vi "CAlex2_Display.vi"(4 "AnkleTraj_Target":dbl[][](array[numeric])=[[0.24613333333333332, -0.7388833333333333, 0.0], [0.24515578259561696, -0.7391742724681776, 0.0], [0.24429789520875214, -0.739459405874052, 0.0], [0.24448752074226363, -0.7393345947088731, 0.0], [0.24469655916514985, -0.7392478031578622, 0.0], [0.24405664388628898, -0.7394239868907534, 0.0], [0.24328071991783762, -0.7396182885443063, 0.0], [0.2423466978742433, -0.7400415973949248, 0.0], [0.24125052807279473, -0.7405823353848426, 0.0], [0.24023250332483256, -0.7409537571683317, 0.0], [0.23967630694566833, -0.7410411536139305, 0.0], [0.2384997454338211, -0.7415221213338982, 0.0], [0.23592724691682573, -0.7427406041862703, 0.0], [0.2344645352495657, -0.7433585608236463, 0.0], [0.2332252795319526, -0.7437143391621577, 0.0], [0.2327208992774311, -0.7438576185144828, 0.0], [0.22915465606710558, -0.7454581765152355, 0.0], [0.2268128238804998, -0.7463847644792208, 0.0], [0.22529565802150417, -0.7469229398096506, 0.0], [0.2250314142391736, -0.7469447859134761, 0.0], [0.22156812672606813, -0.7483363962699071, 0.0], [0.21883255251595407, -0.7494578681789847, 0.0], [0.21756136754091762, -0.7498326608958199, 0.0], [0.2168187315034995, -0.7500358029214264, 0.0], [0.21497895218156837, -0.7506468649505054, 0.0], [0.21286079288286486, -0.7514266489532438, 0.0], [0.21166342103005523, -0.751737076640361, 0.0], [0.21054528432667385, -0.7520154789594069, 0.0], [0.2095433751260343, -0.7522629402601544, 0.0], [0.20845287441942323, -0.752488930880239, 0.0], [0.20742095365351557, -0.752704190462103, 0.0], [0.2051133246644528, -0.753343768184596, 0.0], [0.2038687493698828, -0.7536810637153099, 0.0], [0.2017501089727274, -0.754314257743821, 0.0], [0.19969644651868348, -0.7547514921885444, 0.0], [0.19826758992028087, -0.7551034048067478, 0.0], [0.19615360503043353, -0.7556945908696338, 0.0], [0.19343486835440665, -0.7565103575172124, 0.0], [0.19053313834169708, -0.7574473371460267, 0.0], [0.18843960759791628, -0.7580404798772611, 0.0], [0.18644089773884542, -0.7586060395277501, 0.0], [0.18390809075480052, -0.7594539816458029, 0.0], [0.1808701460626755, -0.7604695651212671, 0.0], [0.17793764820403346, -0.7614543964796003, 0.0], [0.1767810377685385, -0.7618396967115929, 0.0], [0.17456520772270492, -0.7625875498088734, 0.0], [0.17246929355256413, -0.7633236532400511, 0.0], [0.17065935181250597, -0.763955274420301, 0.0], [0.16925675895803116, -0.7643810549322506, 0.0], [0.1685767951889886, -0.7646594472602406, 0.0], [0.16694206859877006, -0.7652765726365656, 0.0], [0.1657034054333985, -0.7656183932135866, 0.0], [0.16450452568282725, -0.7660516442264967, 0.0], [0.1643715030160247, -0.7661069672108636, 0.0], [0.1625504624989272, -0.7667395140519705, 0.0], [0.1616783617927418, -0.7669891645306469, 0.0], [0.16033780666677916, -0.76741690328083, 0.0], [0.16006736860588602, -0.7674978448523857, 0.0], [0.15831402282464435, -0.7680654888349482, 0.0], [0.15675268420907598, -0.768505933121761, 0.0], [0.15526824545197823, -0.7689202252501333, 0.0], [0.1541607197723348, -0.7692489433810146, 0.0], [0.15245036106216156, -0.7696931341913663, 0.0], [0.14957434419557783, -0.7704715732684904, 0.0], [0.14828391270870533, -0.7707643989263094, 0.0], [0.14559288612896337, -0.7714308621646974, 0.0], [0.14439132840557845, -0.7717045322626312, 0.0], [0.1403678029587542, -0.7726695796663579, 0.0], [0.13890481051768733, -0.7729677173493494, 0.0], [0.13575718504559817, -0.7736433469259514, 0.0], [0.1343570726368564, -0.7739458151834464, 0.0], [0.13099009466893163, -0.774589891801166, 0.0], [0.12911814969929047, -0.774937273450445, 0.0], [0.12611842200944545, -0.7754845226684387, 0.0], [0.12384219776075701, -0.7759407221358413, 0.0], [0.12069834992424777, -0.7764745331284479, 0.0], [0.118341694530081, -0.7768570378169698, 0.0], [0.11607436638610731, -0.7772018607169953, 0.0], [0.11314798387040843, -0.7777047090591378, 0.0], [0.11050956015431135, -0.7781152538350306, 0.0], [0.10756675505982971, -0.778548547769883, 0.0], [0.10601252580438528, -0.77874213616469, 0.0], [0.10300893051989053, -0.7791434222500895, 0.0], [0.10059842214669534, -0.7794940247796804, 0.0], [0.09745929116516489, -0.7798971713729205, 0.0], [0.09629140586409997, -0.7800241310447404, 0.0], [0.09332400376079654, -0.780333694859322, 0.0], [0.09103242965898439, -0.7806270861703188, 0.0], [0.08770797963904334, -0.7809774861562493, 0.0], [0.08659441058384258, -0.7810698580287234, 0.0], [0.08426991411154908, -0.7812735166409136, 0.0], [0.0818464656125101, -0.781542090954264, 0.0], [0.07860913641931493, -0.7818772944590949, 0.0], [0.07707091026740395, -0.7820113723411644, 0.0], [0.07555596720741292, -0.7821230905218299, 0.0], [0.07305848865222275, -0.7823716410535728, 0.0], [0.07035157530401719, -0.782669419508252, 0.0], [0.06826387205643206, -0.782862017318102, 0.0], [0.0674716614358491, -0.7829060320001467, 0.0], [0.06506043561731781, -0.7831504929572028, 0.0], [0.06310157689899608, -0.7833812806557202, 0.0], [0.060651473518367305, -0.7836169696991431, 0.0], [0.06010231092573205, -0.7836307056693828, 0.0], [0.05848974929547346, -0.7837615507718494, 0.0], [0.05697455308933186, -0.7839656398243741, 0.0], [0.05464840918973575, -0.7842448590639965, 0.0], [0.05398829908766164, -0.7842628754609134, 0.0], [0.05284711042908441, -0.784307967671166, 0.0], [0.05184067068631544, -0.7844328724163524, 0.0], [0.05004952975847894, -0.7846922419674446, 0.0], [0.04917933101630442, -0.7847515944572329, 0.0], [0.0482067357714643, -0.7847515052312516, 0.0], [0.04700591000093282, -0.784863011448222, 0.0], [0.045323652125186624, -0.78512585869287, 0.0], [0.04441352388868794, -0.7852503533177574, 0.0], [0.04358011009025365, -0.7852037874533097, 0.0], [0.0424444654208676, -0.7852875753729346, 0.0], [0.04126004570310824, -0.7855186232616822, 0.0], [0.040124937873396105, -0.7857250610546572, 0.0], [0.03947411689805993, -0.7856815785943572, 0.0], [0.03845736540920874, -0.7856700898215838, 0.0], [0.037603444107991116, -0.785821981733852, 0.0], [0.03668912531087186, -0.7860330270037836, 0.0], [0.03631201610250871, -0.7860165362475472, 0.0], [0.03522455718085865, -0.7859789899374554, 0.0], [0.03474142561323009, -0.7860480904168305, 0.0], [0.03415715660823453, -0.7862604703380354, 0.0], [0.03381691913063367, -0.7862910817190454, 0.0], [0.03292340364750774, -0.7862265024447485, 0.0], [0.03241768234328942, -0.7862481196110391, 0.0], [0.03202665488082627, -0.7864321951305296, 0.0], [0.03182900463295782, -0.7865167784204048, 0.0], [0.031079149209339147, -0.7864808831658114, 0.0], [0.03038515590143912, -0.7864844060803323, 0.0], [0.030159588775692234, -0.7865929996865106, 0.0], [0.029889439890187133, -0.7867169560834536, 0.0], [0.029348085042040933, -0.7867009127262867, 0.0], [0.028561668290352536, -0.7866845556438959, 0.0], [0.028189689874212, -0.7867619987382084, 0.0], [0.027745017070139672, -0.786942964387257, 0.0], [0.027362567657518766, -0.7869644614468956, 0.0], [0.02638692892411661, -0.7869626934102248, 0.0], [0.026068754674981046, -0.7869979402918131, 0.0], [0.02517144759700583, -0.7872004163901596, 0.0], [0.02477784012412534, -0.7872491344056932, 0.0], [0.02383566271078354, -0.7872600104612801, 0.0], [0.02348938288371493, -0.7872789034032597, 0.0], [0.022213703173392288, -0.7874720576093395, 0.0], [0.021651810632390148, -0.7875615394086567, 0.0], [0.02072286196310254, -0.7875726828739505, 0.0], [0.020294470227114565, -0.7875725727644182, 0.0], [0.019039907077098052, -0.7877057059014416, 0.0], [0.01765463045533501, -0.7878660774364988, 0.0], [0.017008568231705417, -0.7878705475875676, 0.0], [0.016331238534833797, -0.7878674577459974, 0.0], [0.015301524598534443, -0.7879500971410542, 0.0], [0.013175004264126587, -0.7881227684994365, 0.0], [0.012599532933974972, -0.7881362882774775, 0.0], [0.011590794788298088, -0.7881326595475248, 0.0], [0.010982212566540302, -0.7881624877206551, 0.0], [0.008430877492632908, -0.7883089958216887, 0.0], [0.0073701656804433385, -0.7883637054459357, 0.0], [0.006534401238598057, -0.7883369603305339, 0.0], [0.005857106769173521, -0.7883408246568849, 0.0], [0.0036341933158762904, -0.7884203918373144, 0.0], [0.0017199396753864325, -0.7885010154094342, 0.0], [0.001054794556211927, -0.7884804659115676, 0.0], [0.0002567263877230023, -0.7884729911380082, 0.0], [-0.0013181108486029758, -0.7884919168187614, 0.0], [-0.004009114624084201, -0.7885646159414788, 0.0], [-0.004721619017951035, -0.788563571578087, 0.0], [-0.005490707534985728, -0.7885368856950778, 0.0], [-0.006720271622264472, -0.7885221798013166, 0.0], [-0.00946256190968962, -0.7885426790574998, 0.0], [-0.0107773510970461, -0.7885526806198543, 0.0], [-0.011404177158667525, -0.7885254499937199, 0.0], [-0.01230370632954732, -0.7885099737771037, 0.0], [-0.014783720031384435, -0.788505360160213, 0.0], [-0.016655495616472324, -0.7885000050444746, 0.0], [-0.017352058861391, -0.7884684140217153, 0.0], [-0.01801104065566522, -0.7884278820318243, 0.0], [-0.020159474340736516, -0.7883818273511758, 0.0], [-0.022198356752492057, -0.7883834862202718, 0.0], [-0.023377406887171867, -0.7883564009689698, 0.0], [-0.023715126260462696, -0.7883258761914703, 0.0], [-0.02546803605106259, -0.7882808163999377, 0.0], [-0.02764678331393335, -0.7882522527772768, 0.0], [-0.02900583751499738, -0.7882179655472195, 0.0], [-0.029503264776825258, -0.7881835478310103, 0.0], [-0.030670043396237794, -0.7881356235738904, 0.0], [-0.03290540286290335, -0.7880696389206449, 0.0], [-0.03424051453549059, -0.7880319431567786, 0.0], [-0.03518867698164292, -0.7879865813917275, 0.0], [-0.035708520712345156, -0.7879516963423487, 0.0], [-0.03785604851305007, -0.7878534552815656, 0.0], [-0.039173831000815784, -0.7878079902289162, 0.0], [-0.04031305495094807, -0.7877480464957666, 0.0], [-0.040775374063418565, -0.7877090222363465, 0.0], [-0.042371807747924595, -0.7876329980068867, 0.0], [-0.04390308424613412, -0.7875610592614354, 0.0], [-0.044893376222619144, -0.7875144179579441, 0.0], [-0.04564564925107059, -0.7874679571001013, 0.0], [-0.04656707813226394, -0.7874055062676626, 0.0], [-0.04824029119510185, -0.7872916822301301, 0.0], [-0.04904894550139232, -0.7872516191181922, 0.0], [-0.05000363023846826, -0.7871794139623552, 0.0], [-0.05069263439155017, -0.7871412478324679, 0.0], [-0.05202764767163273, -0.7870474284270107, 0.0], [-0.05298811443341366, -0.7869667161446681, 0.0], [-0.053770878548014114, -0.7868941577787267, 0.0], [-0.05459432155515526, -0.7868264205955833, 0.0], [-0.055461819619422065, -0.7867529685001882, 0.0], [-0.056634066465346904, -0.7866465700876712, 0.0], [-0.057223819714484835, -0.7865958266471488, 0.0], [-0.05822818983782874, -0.7864995542146789, 0.0], [-0.05888556085452924, -0.7864434159578955, 0.0], [-0.05997878318995532, -0.786336537681881, 0.0], [-0.060747251544050335, -0.7862651717599778, 0.0], [-0.06154929157510758, -0.7861805478817437, 0.0], [-0.06238461562291835, -0.7860944181250622, 0.0], [-0.06321052646340114, -0.7860077538688077, 0.0], [-0.06431083300249688, -0.7858786867171308, 0.0], [-0.0649946346567653, -0.7858022812056326, 0.0], [-0.06597802816340989, -0.7856949410158913, 0.0], [-0.06663767976420029, -0.7856173886891471, 0.0], [-0.06795606111781928, -0.7854548450334109, 0.0], [-0.06885321364907762, -0.785351471611811, 0.0], [-0.06967376061251168, -0.7852434997192976, 0.0], [-0.0706422839266972, -0.7851287975124323, 0.0], [-0.07166185154535253, -0.7850070449374327, 0.0], [-0.07320001399122117, -0.7848166996970609, 0.0], [-0.07366284492618107, -0.7847477237306885, 0.0], [-0.07509107248592095, -0.7845846675065444, 0.0], [-0.07573304869493647, -0.7844933210836742, 0.0], [-0.07783852524090834, -0.7841811413409909, 0.0], [-0.07830638873019802, -0.784113816047286, 0.0], [-0.07986142248668965, -0.7839136830476261, 0.0], [-0.08057983843469357, -0.7838133611250357, 0.0], [-0.08254712925686795, -0.7835107319583848, 0.0], [-0.08372130434764231, -0.7833332506546589, 0.0], [-0.08487482140537983, -0.783178322028624, 0.0], [-0.08624135215637413, -0.7830037405553079, 0.0], [-0.08748571040426449, -0.7827962829871418, 0.0], [-0.0895638539320319, -0.7824591761767064, 0.0], [-0.09033022919915192, -0.7823437713500916, 0.0], [-0.09223469613748583, -0.7820558585723796, 0.0], [-0.09303631599513518, -0.7819242041034085, 0.0], [-0.09537564242715288, -0.7814955495412113, 0.0], [-0.09647386843985803, -0.781298844845439, 0.0], [-0.0983505446047384, -0.7809952024764676, 0.0], [-0.09939197545609449, -0.7808303999018062, 0.0], [-0.10117703859613394, -0.780479144010592, 0.0], [-0.10307739897768062, -0.7801058716544537, 0.0], [-0.10458410669158132, -0.7798233513601808, 0.0], [-0.10631614948309831, -0.7795040320845944, 0.0], [-0.10724061359126007, -0.7793124203492745, 0.0], [-0.1098252331880692, -0.7787507023360662, 0.0], [-0.11118802584963487, -0.7784571826812104, 0.0], [-0.1134401070088136, -0.7780001641140143, 0.0], [-0.11398997768348407, -0.7778998615960213, 0.0], [-0.1164778575110416, -0.7772996866609776, 0.0], [-0.1181717940663653, -0.7768863467573213, 0.0], [-0.12066860475959379, -0.7763223189444195, 0.0], [-0.1214141962112577, -0.7761766991536709, 0.0], [-0.12324044731997584, -0.7756735262994104, 0.0], [-0.1254773206809978, -0.7750478230549499, 0.0], [-0.1278924360774777, -0.7744240727286277, 0.0], [-0.12921853695853153, -0.7741273427918501, 0.0], [-0.13026599200310643, -0.7738321755872171, 0.0], [-0.1328264905613512, -0.7730393629477945, 0.0], [-0.13517221445668215, -0.772357930314364, 0.0], [-0.13720511623991974, -0.7718098114576666, 0.0], [-0.13770659806181337, -0.771675739116628, 0.0], [-0.1401844389971911, -0.7708316127409436, 0.0], [-0.14248754289563006, -0.7700929873871858, 0.0], [-0.14503768099654107, -0.769289278577148, 0.0], [-0.14557750618101167, -0.7691803977996958, 0.0], [-0.14746986736043616, -0.7684261182538246, 0.0], [-0.14991232932304877, -0.7675411849979178, 0.0], [-0.1525093218513537, -0.7666150255659575, 0.0], [-0.15352826964278496, -0.7663174796823413, 0.0], [-0.15462071853739745, -0.7658054188771892, 0.0], [-0.1572225876287715, -0.7647397773653982, 0.0], [-0.15956896179024835, -0.7638012789023148, 0.0], [-0.16118181666413148, -0.7631848529453348, 0.0], [-0.1617132790024308, -0.7629132233699157, 0.0], [-0.16400798872387004, -0.7617854289722976, 0.0], [-0.16614694592442525, -0.7608493885441028, 0.0], [-0.16794638606264142, -0.7599932650782975, 0.0], [-0.1683225857071199, -0.759779362579468, 0.0], [-0.1699769170071399, -0.7587593491288297, 0.0], [-0.17186490276842684, -0.7577711398641326, 0.0], [-0.17349617867901543, -0.7567964031229927, 0.0], [-0.17392368788780974, -0.7564718113150823, 0.0], [-0.17491070255363497, -0.7556716244470942, 0.0], [-0.17651750620363071, -0.7545597916249724, 0.0], [-0.17799167744774833, -0.7535190397566246, 0.0], [-0.17833649143631383, -0.7530393693379724, 0.0], [-0.1787408329455695, -0.7524603471010285, 0.0], [-0.18000418295968346, -0.751238706857306, 0.0], [-0.18145315127794903, -0.7500681251432028, 0.0], [-0.1816559576043227, -0.7494557656604731, 0.0], [-0.1816644212975711, -0.7489644437811844, 0.0], [-0.1823317455763194, -0.7478734173226511, 0.0], [-0.18384316588694824, -0.7464202083479551, 0.0], [-0.18401787835473926, -0.7456367975833745, 0.0], [-0.18361681682665348, -0.7451773148747894, 0.0], [-0.18364861997236692, -0.7443345459824955, 0.0], [-0.185062660884808, -0.7426564755347907, 0.0], [-0.18560288443037376, -0.7415908164436046, 0.0], [-0.1846870880509903, -0.7411675941367387, 0.0], [-0.1842413522530071, -0.7404925571045282, 0.0], [-0.1850925285936018, -0.738872432044968, 0.0], [-0.18616201229315876, -0.7373470443283474, 0.0], [-0.18496317306601276, -0.7349003633464255, 0.0], [-0.18387215151573422, -0.7325775861892544, 0.0], [-0.18410094359418533, -0.7316757672054778, 0.0], [-0.18535803931122757, -0.7316853596407139, 0.0], [-0.18446035631468438, -0.7297804799503158, 0.0], [-0.18249453490739878, -0.7261884991854444, 0.0], [-0.18229756232106015, -0.725136432724723, 0.0], [-0.1833521987739792, -0.7242580631619052, 0.0], [-0.18309058984192675, -0.723250177106378, 0.0], [-0.18045672952710184, -0.7189719165546526, 0.0], [-0.17972191205538401, -0.7175610692159828, 0.0], [-0.18047955032563326, -0.716229914823051, 0.0], [-0.18070712580575254, -0.7153915855745955, 0.0], [-0.17825379959787585, -0.7119444492952096, 0.0], [-0.17660541271202532, -0.7095829787048227, 0.0], [-0.17726836299409499, -0.70863141238353, 0.0], [-0.17756465634286484, -0.7071043860892063, 0.0], [-0.17597388752858023, -0.7052396472805906, 0.0], [-0.1735067428811073, -0.7021023572741115, 0.0], [-0.17395262277216852, -0.7015874825495777, 0.0], [-0.17431227109386013, -0.6996327073293189, 0.0], [-0.17351098959655947, -0.6987013188789766, 0.0], [-0.17090905634883544, -0.6956975759194545, 0.0], [-0.17071526899782985, -0.6949628916533201, 0.0], [-0.1710730978739466, -0.6932998549428917, 0.0], [-0.17059969366613145, -0.6922655001854908, 0.0], [-0.1685086096213139, -0.6902548267595341, 0.0], [-0.16756778617430831, -0.6888452218007766, 0.0], [-0.16783904554105128, -0.6879094949373579, 0.0], [-0.16744372710126487, -0.6864135750864528, 0.0], [-0.16607676729082885, -0.6854063822431189, 0.0], [-0.16428868333505256, -0.6834491190056624, 0.0], [-0.16437288207930492, -0.6829889256346043, 0.0], [-0.1635520369623697, -0.6813633896985897, 0.0], [-0.1628656444125077, -0.6808215511725021, 0.0], [-0.16064844714157672, -0.6790265874442762, 0.0], [-0.16025039941082478, -0.6784939238787473, 0.0], [-0.15901464757812167, -0.6774100829862024, 0.0], [-0.15838258213735087, -0.6768209547329185, 0.0], [-0.156403180343882, -0.6756546958660214, 0.0], [-0.1551046893102324, -0.6748992410569326, 0.0], [-0.15378650496489113, -0.674475626863044, 0.0], [-0.15243497736837558, -0.6740336347150155, 0.0], [-0.15104960487783037, -0.673376061060042, 0.0], [-0.14895742655204294, -0.6727337874919133, 0.0], [-0.14752407158209987, -0.6726148951231982, 0.0], [-0.14552447065928026, -0.6727450331083875, 0.0], [-0.14413685156931189, -0.6723830485253336, 0.0], [-0.14201185621486456, -0.6719499124071664, 0.0], [-0.13999712302609457, -0.6719010844966414, 0.0], [-0.13789764232007043, -0.6724575196088171, 0.0], [-0.13581766368011372, -0.6724792988084772, 0.0], [-0.1341221643754686, -0.6721198120451769, 0.0], [-0.1314855746330025, -0.6720108651382866, 0.0], [-0.12929049312761973, -0.672756136444688, 0.0], [-0.126557754314033, -0.6732133304526884, 0.0], [-0.12489632665279873, -0.6730547887078726, 0.0], [-0.12234428885258374, -0.6727813448644856, 0.0], [-0.11981886787835304, -0.6735674837877927, 0.0], [-0.11687430283673697, -0.6743997481810158, 0.0], [-0.11463236714075, -0.6746290428943977, 0.0], [-0.11242247503721689, -0.674244134280172, 0.0], [-0.10953774192295711, -0.6749858199504095, 0.0], [-0.10622097062492893, -0.6761232107744019, 0.0], [-0.10351434067614276, -0.6767183066919363, 0.0], [-0.10138526967839516, -0.676419229068994, 0.0], [-0.0987453833688493, -0.6769263701238192, 0.0], [-0.09495904699190161, -0.6782958725667444, 0.0], [-0.0919303847353094, -0.6792138083547098, 0.0], [-0.0894125143219684, -0.6792359514227291, 0.0], [-0.0871375322538299, -0.6794833204561684, 0.0], [-0.0831215330763308, -0.6809377595726507, 0.0], [-0.07957563610649226, -0.6821650323344924, 0.0], [-0.07687887623091821, -0.6824561680643375, 0.0], [-0.07457374418393287, -0.6827041585258318, 0.0], [-0.07083498058370374, -0.6840153647832246, 0.0], [-0.06657030782438772, -0.6855689187674324, 0.0], [-0.06378688721473509, -0.6860762337057521, 0.0], [-0.06133856452416751, -0.6864470563027192, 0.0], [-0.05791458688631438, -0.6875212491094306, 0.0], [-0.053455723210862297, -0.6891942292569727, 0.0], [-0.04992107855511799, -0.690129800915217, 0.0], [-0.04785976548703769, -0.6904687897635167, 0.0], [-0.04429650378985464, -0.691505403605125, 0.0], [-0.040267513266939975, -0.6930072731511884, 0.0], [-0.03555784713241386, -0.6944672859111183, 0.0], [-0.033952270770763925, -0.6947575304830064, 0.0], [-0.030294611985942483, -0.6957952014736306, 0.0], [-0.026730238455901584, -0.6969952577065013, 0.0], [-0.021509173930342365, -0.6987415905159186, 0.0], [-0.019147837592746794, -0.6994085909252956, 0.0], [-0.016465655647499366, -0.7000922265796167, 0.0], [-0.012615180760201874, -0.7012186563230334, 0.0], [-0.007974830010891241, -0.7027641525791309, 0.0], [-0.0038514626540264224, -0.7041578766964204, 0.0], [-0.0024991707475486144, -0.7044355441470568, 0.0], [0.001713991955020735, -0.7055298202171897, 0.0], [0.005467445940488787, -0.7067174714149304, 0.0], [0.011086793879152207, -0.7086648050804788, 0.0], [0.012346067696271603, -0.7090082450295017, 0.0], [0.015624141185188893, -0.709686955311302, 0.0], [0.01949821698524377, -0.7107804212528472, 0.0], [0.025228550445434386, -0.7127347621775503, 0.0], [0.028095178501171585, -0.7136763319986967, 0.0], [0.029577853817759465, -0.7137674373694146, 0.0], [0.03402213615239169, -0.714855026809285, 0.0], [0.03890264621843478, -0.7164824758991323, 0.0], [0.04401630068690935, -0.7181206210901309, 0.0], [0.044150665343611936, -0.7179077692705919, 0.0], [0.04850409059409398, -0.7187915624395463, 0.0], [0.052826849085273984, -0.7201520956830715, 0.0], [0.05936157438052341, -0.7221317572745819, 0.0], [0.0598606923988813, -0.7221604140593466, 0.0], [0.06280990854294137, -0.7225980552566091, 0.0], [0.0672636510917792, -0.723832004285925, 0.0], [0.07378549322636403, -0.7256628814422235, 0.0], [0.07614007746049441, -0.7262339999817666, 0.0], [0.07739123386413825, -0.7262856621210743, 0.0], [0.08180173412478348, -0.7273335805255913, 0.0], [0.08768398411078117, -0.7288428313495438, 0.0], [0.09216893731751477, -0.729894959133162, 0.0], [0.09274421254028138, -0.7298836209866717, 0.0], [0.09637643378246555, -0.7306779131751931, 0.0], [0.1014618726263282, -0.7318058486357247, 0.0], [0.10723393364075276, -0.7330366292260817, 0.0], [0.10840815416195484, -0.73322556772305, 0.0], [0.11099695176226294, -0.7338048959190883, 0.0], [0.11515688377075128, -0.7346212018501824, 0.0], [0.12116830930064156, -0.7356724472145532, 0.0], [0.12391878867444962, -0.7361952029478482, 0.0], [0.1258724199892303, -0.7366183213350824, 0.0], [0.129017903497053, -0.737262113559882, 0.0], [0.13413748208308635, -0.737901286006338, 0.0], [0.13867311213960196, -0.73867403275472, 0.0], [0.14059053613570796, -0.7390290288960936, 0.0], [0.1429520240087575, -0.7395939766676461, 0.0], [0.14647218801328787, -0.7399149183300441, 0.0], [0.15202509874676606, -0.7406121467389591, 0.0], [0.1548313416916139, -0.7410619688502749, 0.0], [0.1566217943097276, -0.741469966748341, 0.0], [0.1587066676086444, -0.7417244974470258, 0.0], [0.16363434193410317, -0.7420513953005045, 0.0], [0.1681251634394015, -0.7426462555691024, 0.0], [0.16956603316542496, -0.7428640773389403, 0.0], [0.17091249419614715, -0.7432205234759091, 0.0], [0.17385061646281466, -0.7432314686630598, 0.0], [0.1798623393445299, -0.7437692679464494, 0.0], [0.1816278843383637, -0.7438484666245391, 0.0], [0.18277371258129246, -0.7442452051872732, 0.0], [0.18373056032093663, -0.7442434120363641, 0.0], [0.18970100653697647, -0.7444762536345672, 0.0], [0.19282515627076582, -0.7444792886102092, 0.0], [0.19389190526009192, -0.7447248030952623, 0.0], [0.1940024622438909, -0.7448954687296633, 0.0], [0.198268381339083, -0.7448860217837132, 0.0], [0.203256183772467, -0.7447528318726716, 0.0], [0.2042820203198384, -0.7447990161681439, 0.0], [0.20457696796778815, -0.7450598025228328, 0.0], [0.206179703507099, -0.7450912809560972, 0.0], [0.21124441886523704, -0.7448144753282405, 0.0], [0.21296257849351108, -0.7446553786860197, 0.0], [0.21350847568633377, -0.7448613546951254, 0.0], [0.21356452837855547, -0.7450557300400247, 0.0], [0.21756060282016337, -0.7446462276242277, 0.0], [0.2205637818546301, -0.7442697674937395, 0.0], [0.2214850252667741, -0.7442890153122755, 0.0], [0.2210344078232337, -0.7446045213100679, 0.0], [0.22294049697804816, -0.7442931127256188, 0.0], [0.22681850164500902, -0.7436409161299977, 0.0], [0.22835262368996143, -0.7434430260745569, 0.0], [0.22806876482098565, -0.7437359686242714, 0.0], [0.22797651032722144, -0.74373031602662, 0.0], [0.23159506581956135, -0.7429820682623874, 0.0], [0.23389945600596412, -0.7424902363950557, 0.0], [0.23404227959254578, -0.7425922016496063, 0.0], [0.2325256549614945, -0.7428880401951851, 0.0], [0.2375025139378799, -0.7417892959296368, 0.0], [0.24160373313665298, -0.7408549700233856, 0.0], [0.2418966425051684, -0.7408258524796333, 0.0], [0.2405339902575081, -0.7410767675787858, 0.0], [0.24117268995111793, -0.7408384164749444, 0.0], [0.24414060397165194, -0.7400216235559133, 0.0], [0.2453596754941961, -0.7397383404869367, 0.0], [0.24412705505999177, -0.7399090785004065, 0.0], [0.24347014810519474, -0.7399890635784795, 0.0], [0.2452444444444445, -0.7394555555555555, 0.0]], 5 "ClosePt":dbl[](array[numeric]), 6 "Init?":bool, 7 "Field Force":dbl[](array[numeric]), 8 "error in (no error)":errorcluster, 9 "AxisSetting":T1={"AxisLabel"=["x ", "y", "z "], "AxisMax"=[0.6, 0.7, 0.2], "AxisMin"=[-0.4, -0.3, -0.8]}, 10 "3D graph in":refnum<k7>, 11 "CLX2 in":refnum<class "CAlex2_Display.lvclass">) -> (0 "error out":errorcluster, 1 "LastPlotNum":i32=1, 2 "3D graph out":refnum<k7>, 3 "CLX2 out":refnum<class "CAlex2_Display.lvclass">)   [LabVIEW 2016, in "CAlex2_Display.lvclass"]
uses:
  CAlex2_Display.lvclass
  D:/JinXin/LabVIEW.git/CAlex2-Controller-mobile/Classes/SerialChain/SerialChain.lvclass
  D:/JinXin/LabVIEW.git/CAlex2-Controller-mobile/Classes/SerialChain-Cable/SerialChain-Cable.lvclass
  <vilib>/Platform/NI_3dgraph.lvlib
  <vilib>/ptbypt/NI_PtbyPt.lvlib
  SerialChain/SerialChain.lvclass
  SerialChain-Cable/SerialChain-Cable.lvclass
panel:
  out "EndEffInGCS":dbl[](array[numeric]) format="%#.6f"
  in  "sample length":i32=15
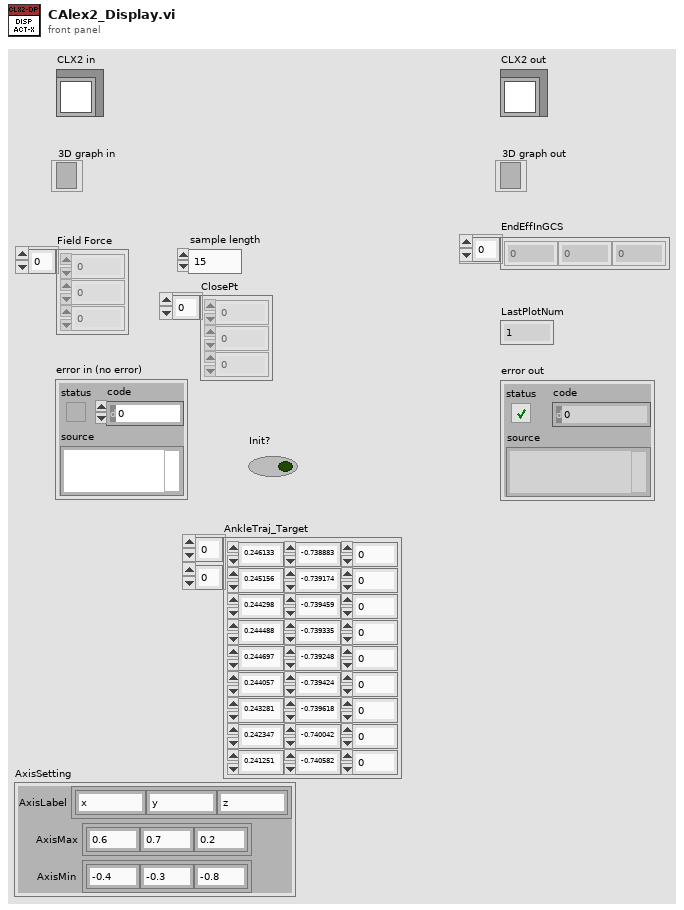
[diagram p1: front panel]
types:
  T1 = cluster{"AxisLabel":string[], "AxisMax":dbl[], "AxisMin":dbl[]}
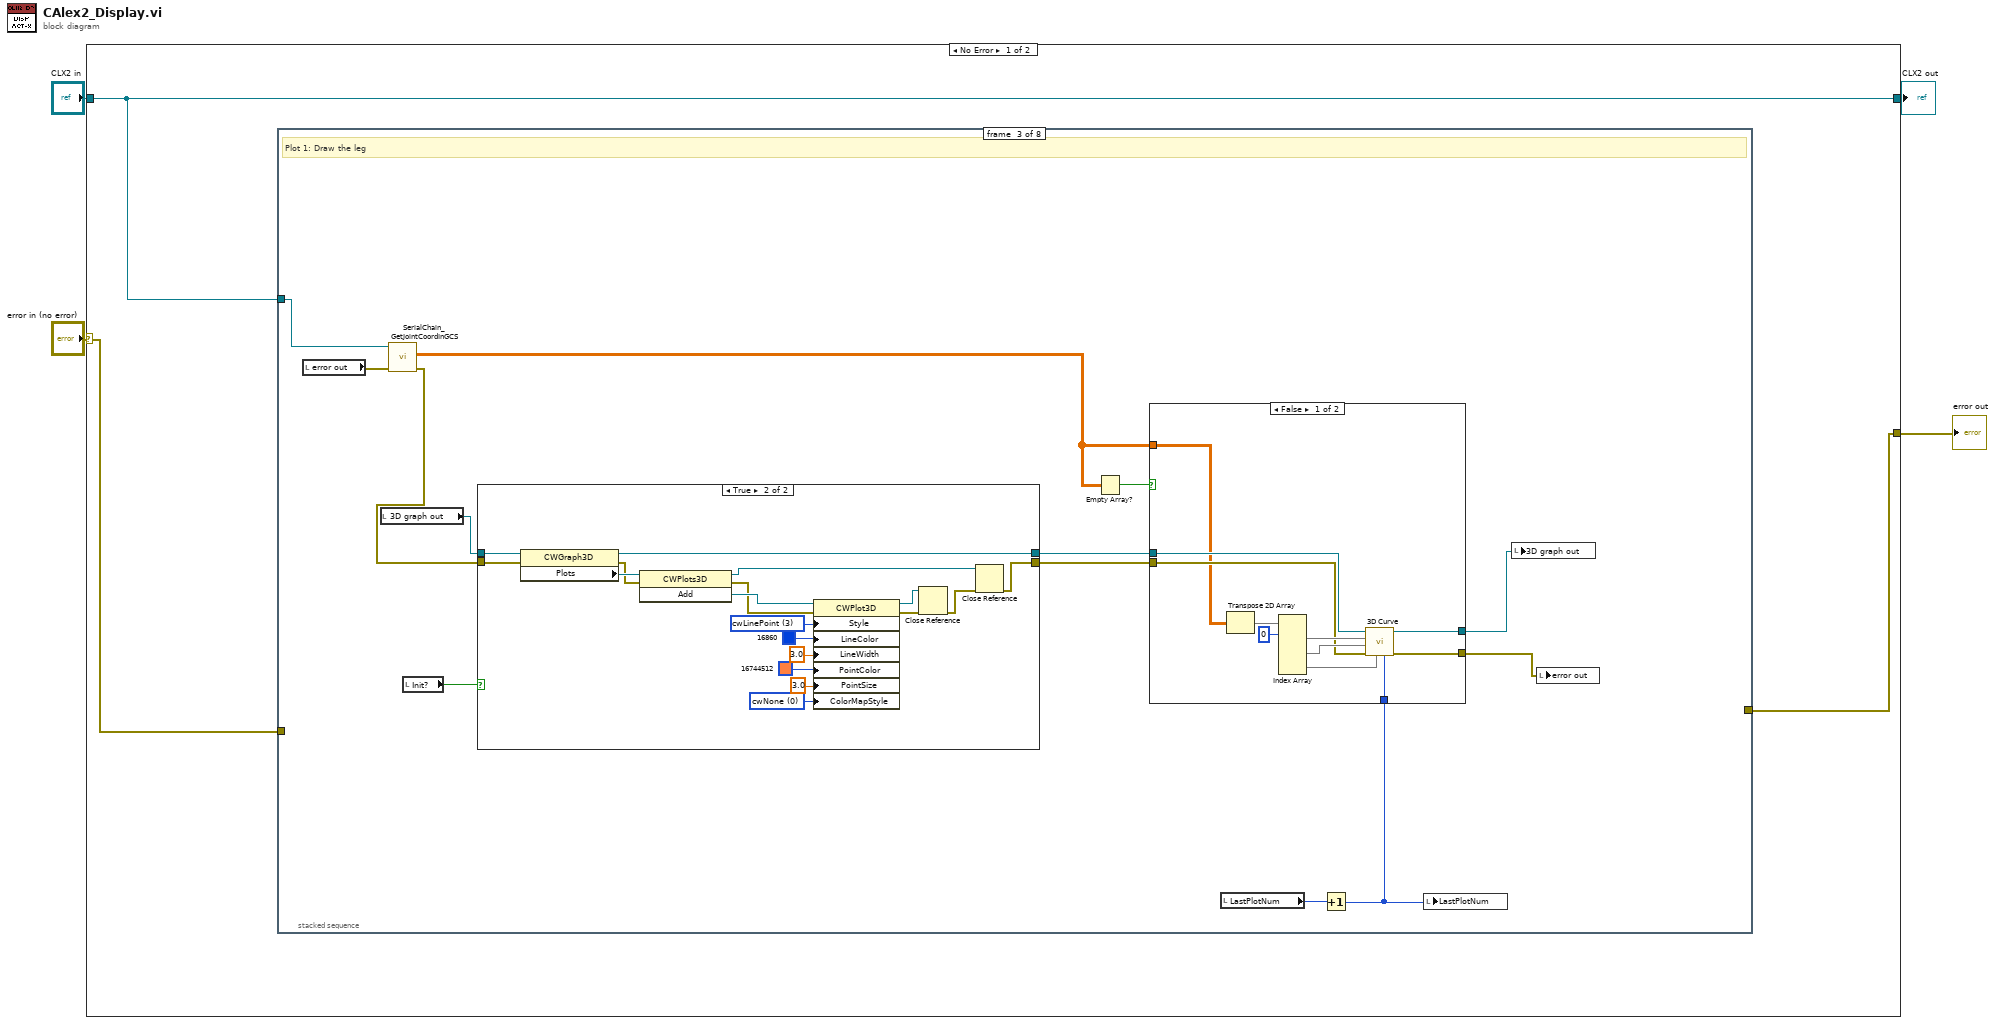
[diagram p0: block diagram]
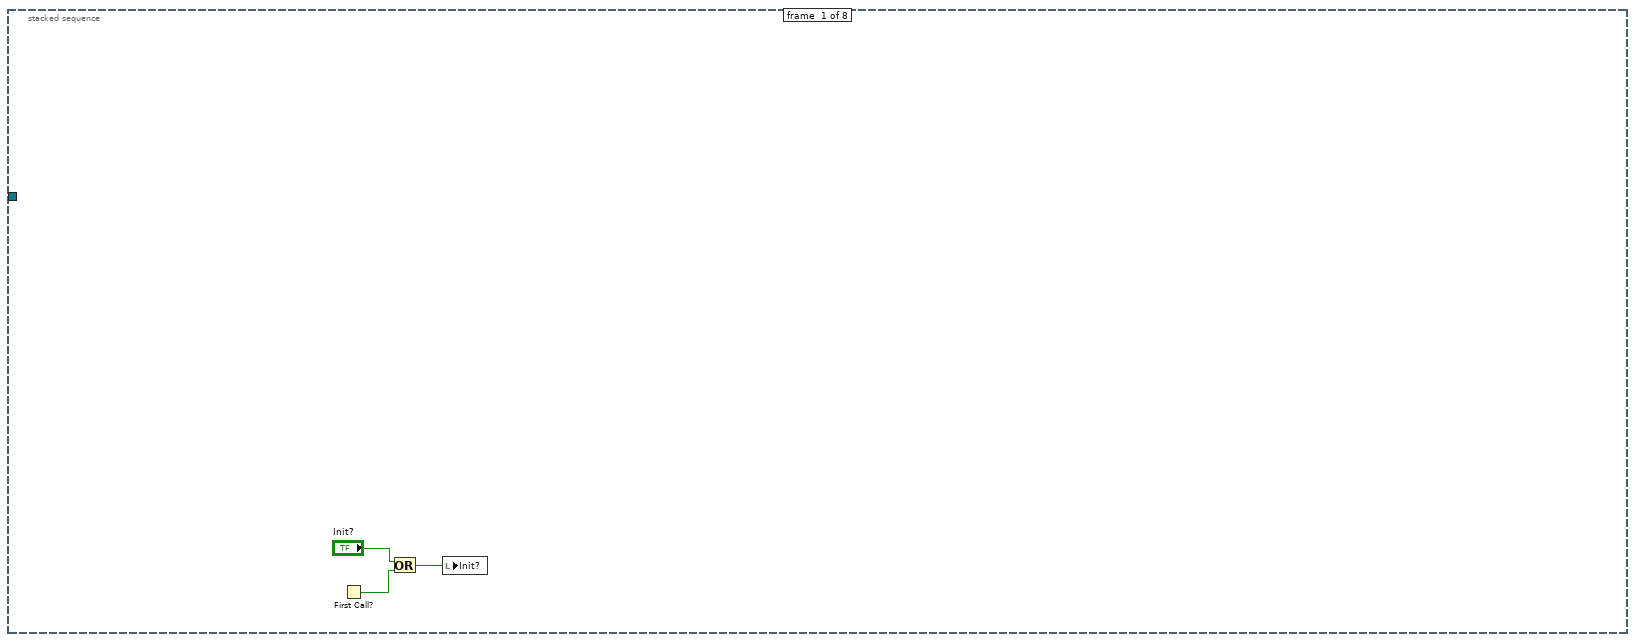
[diagram p2: hidden frame]
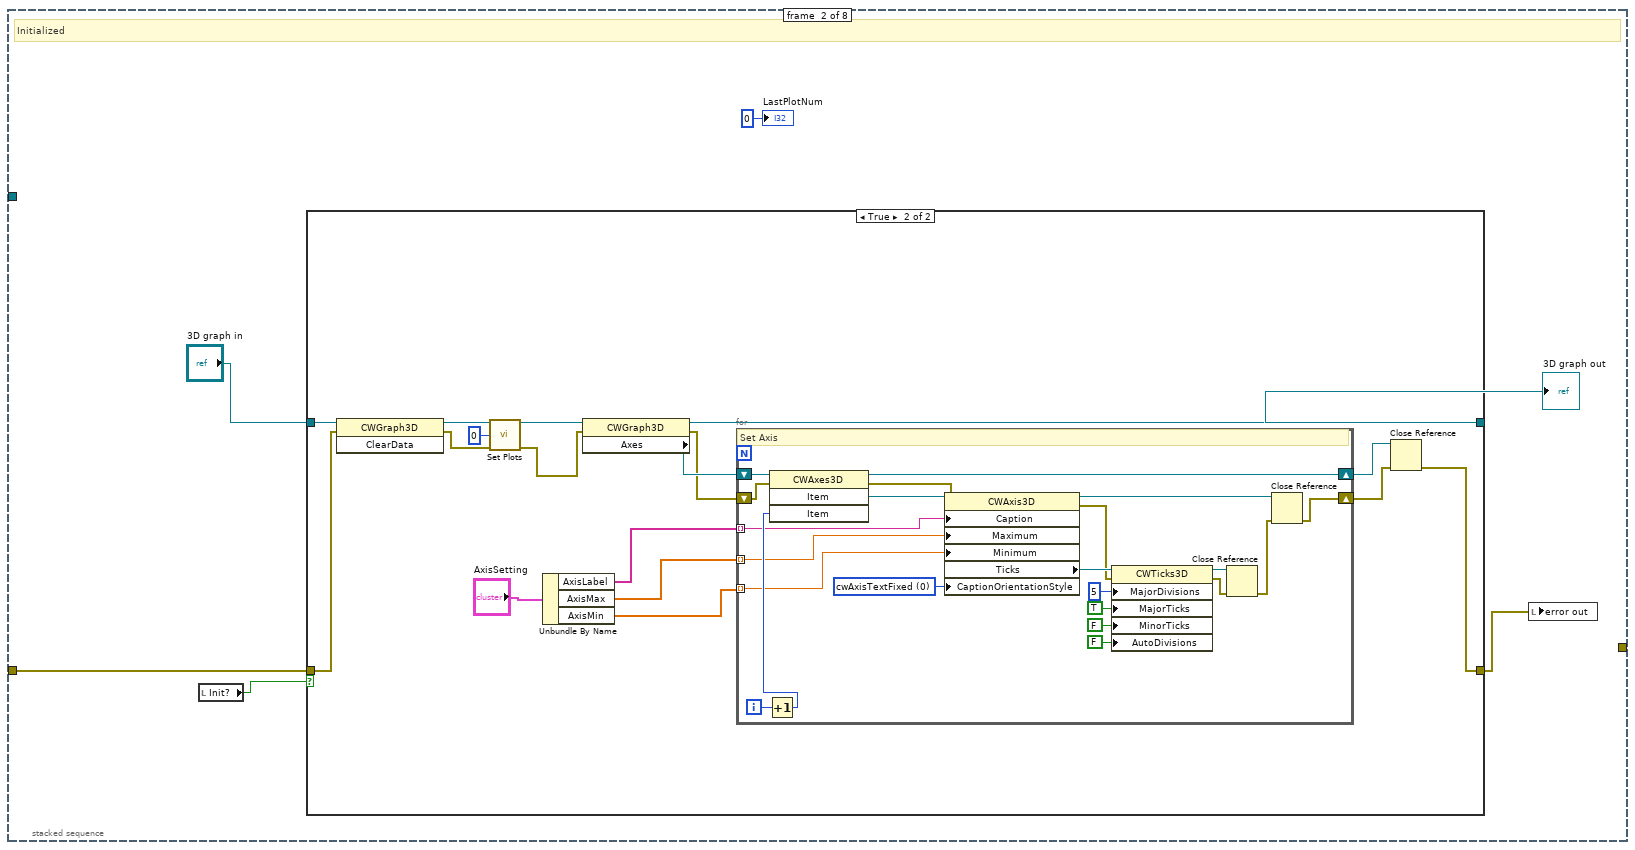
[diagram p3: hidden frame]
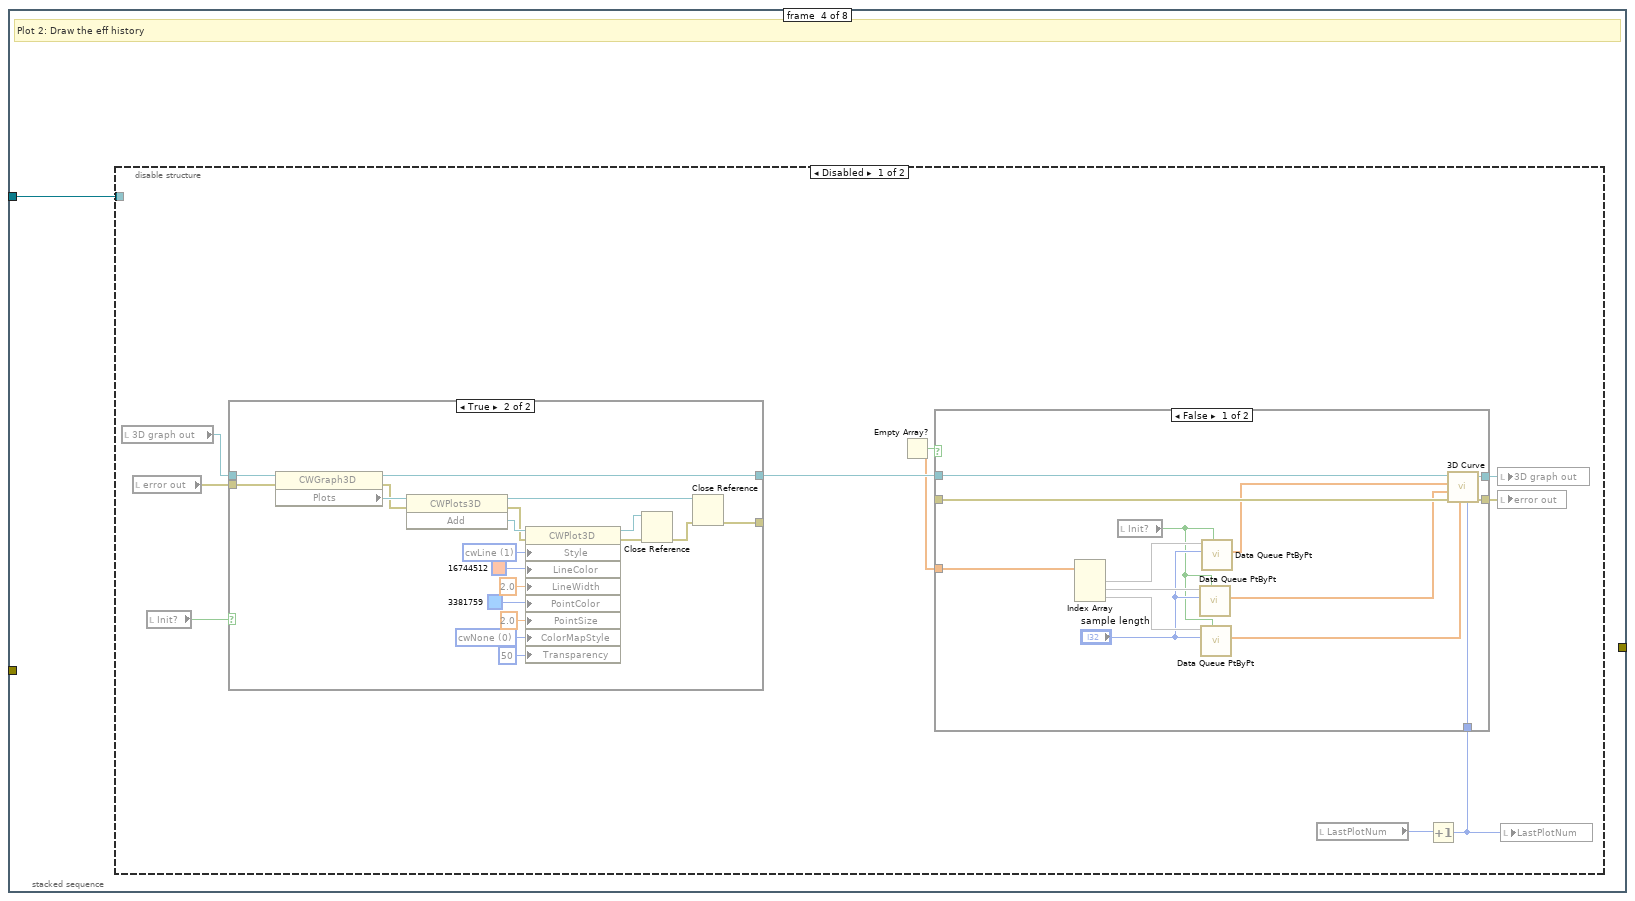
[diagram p7: hidden frame]
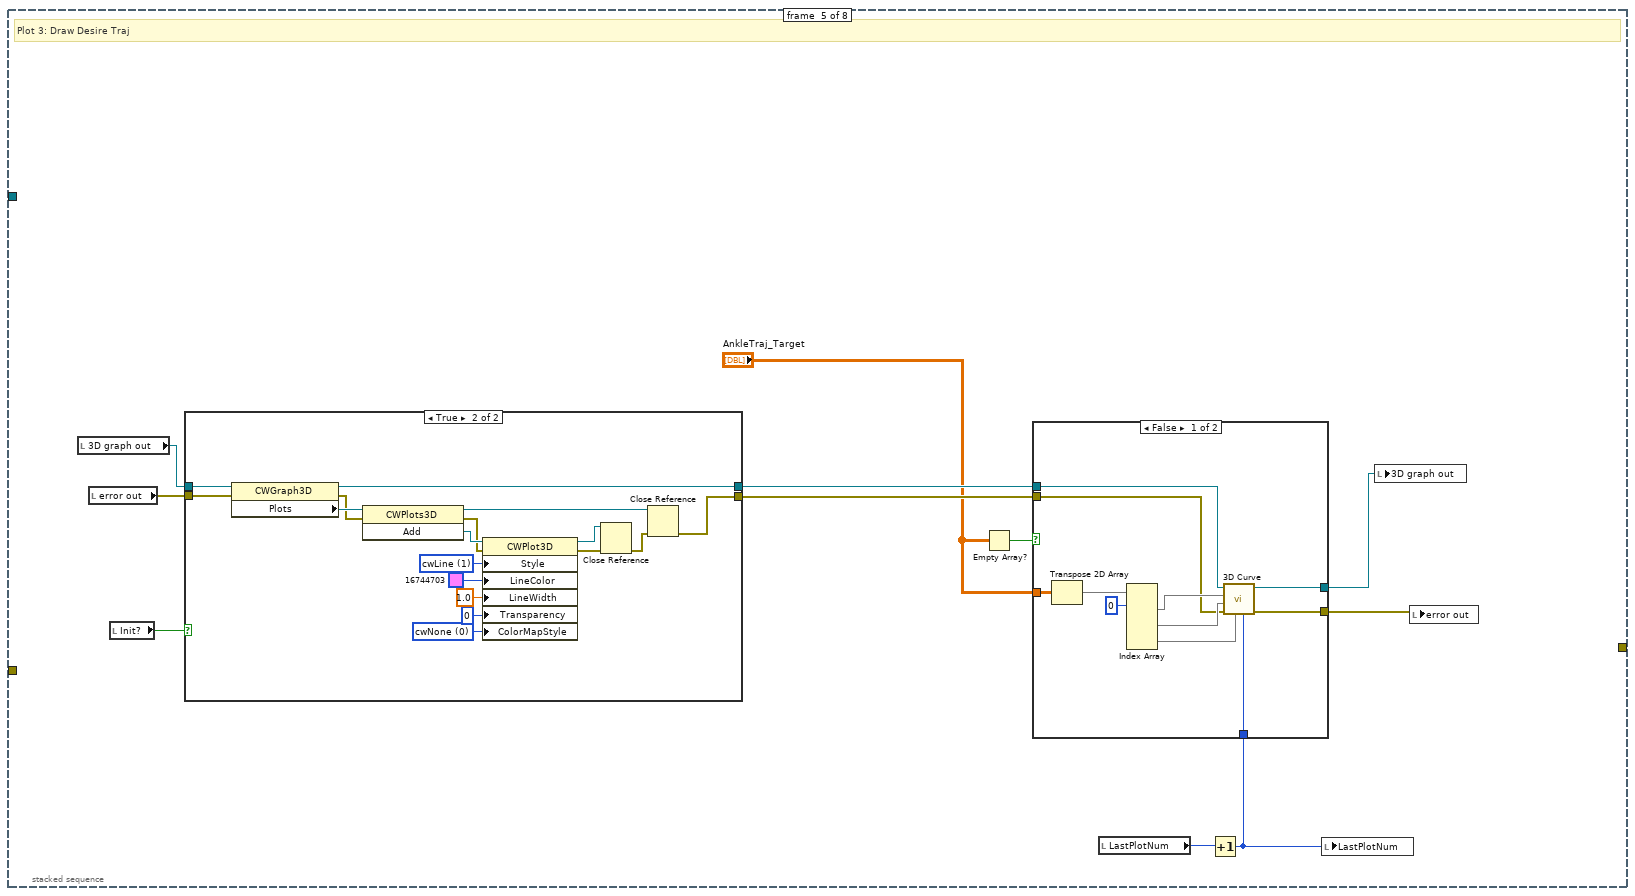
[diagram p11: hidden frame]
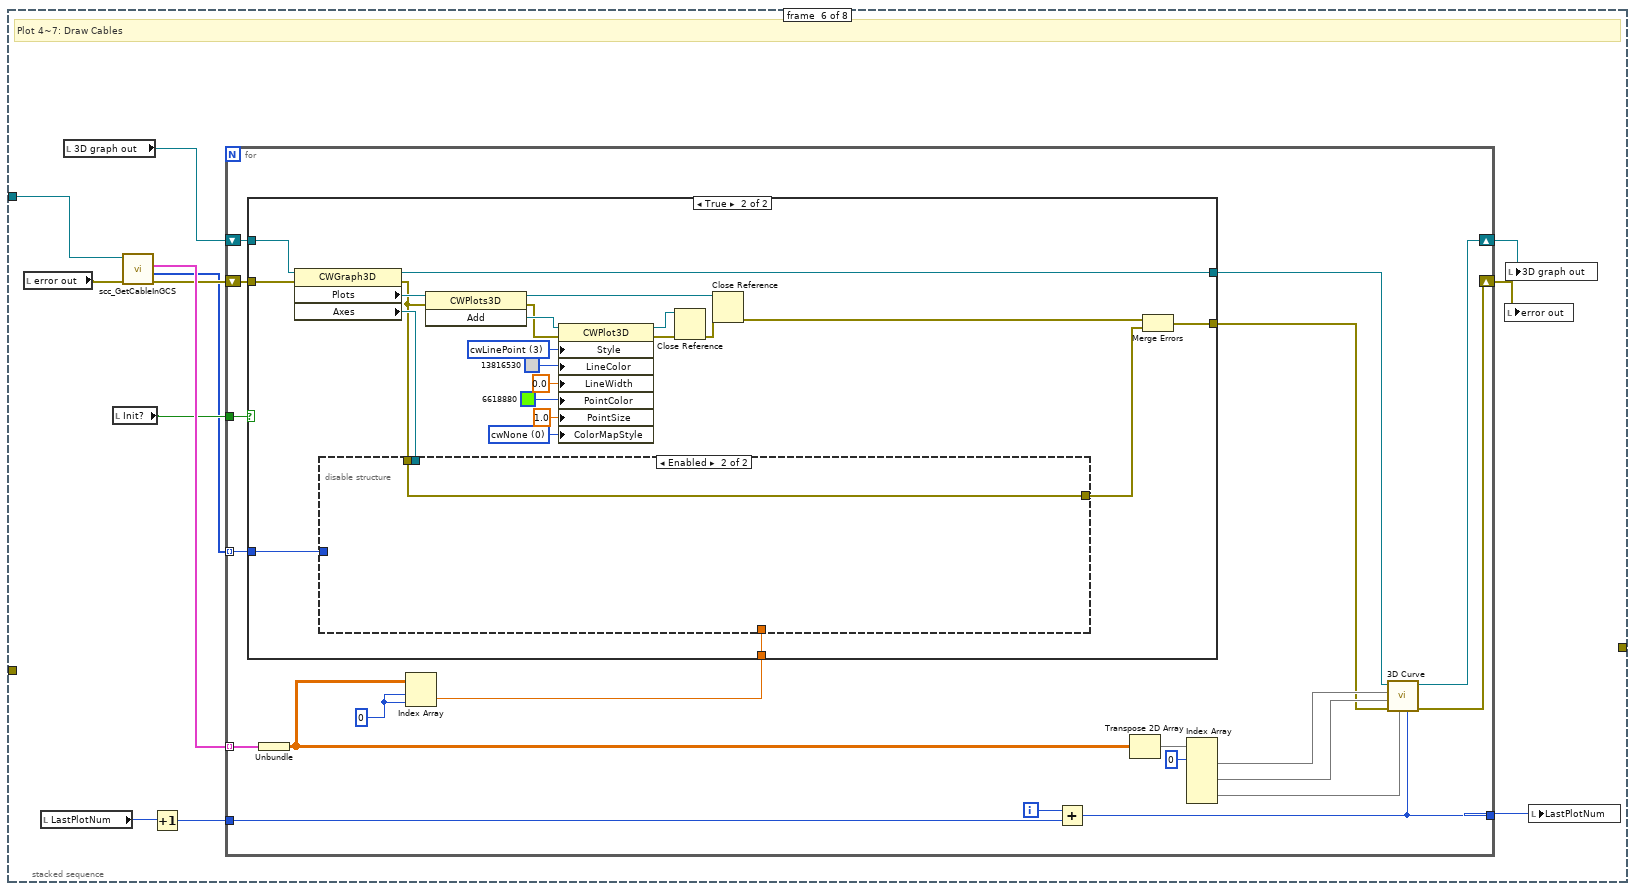
[diagram p14: hidden frame]
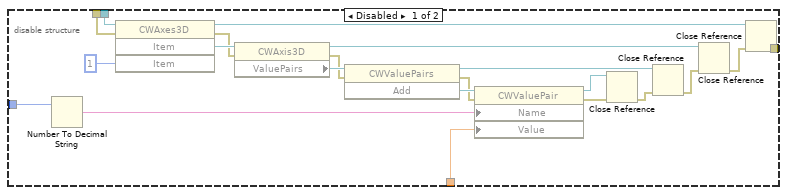
[diagram p16: hidden frame]
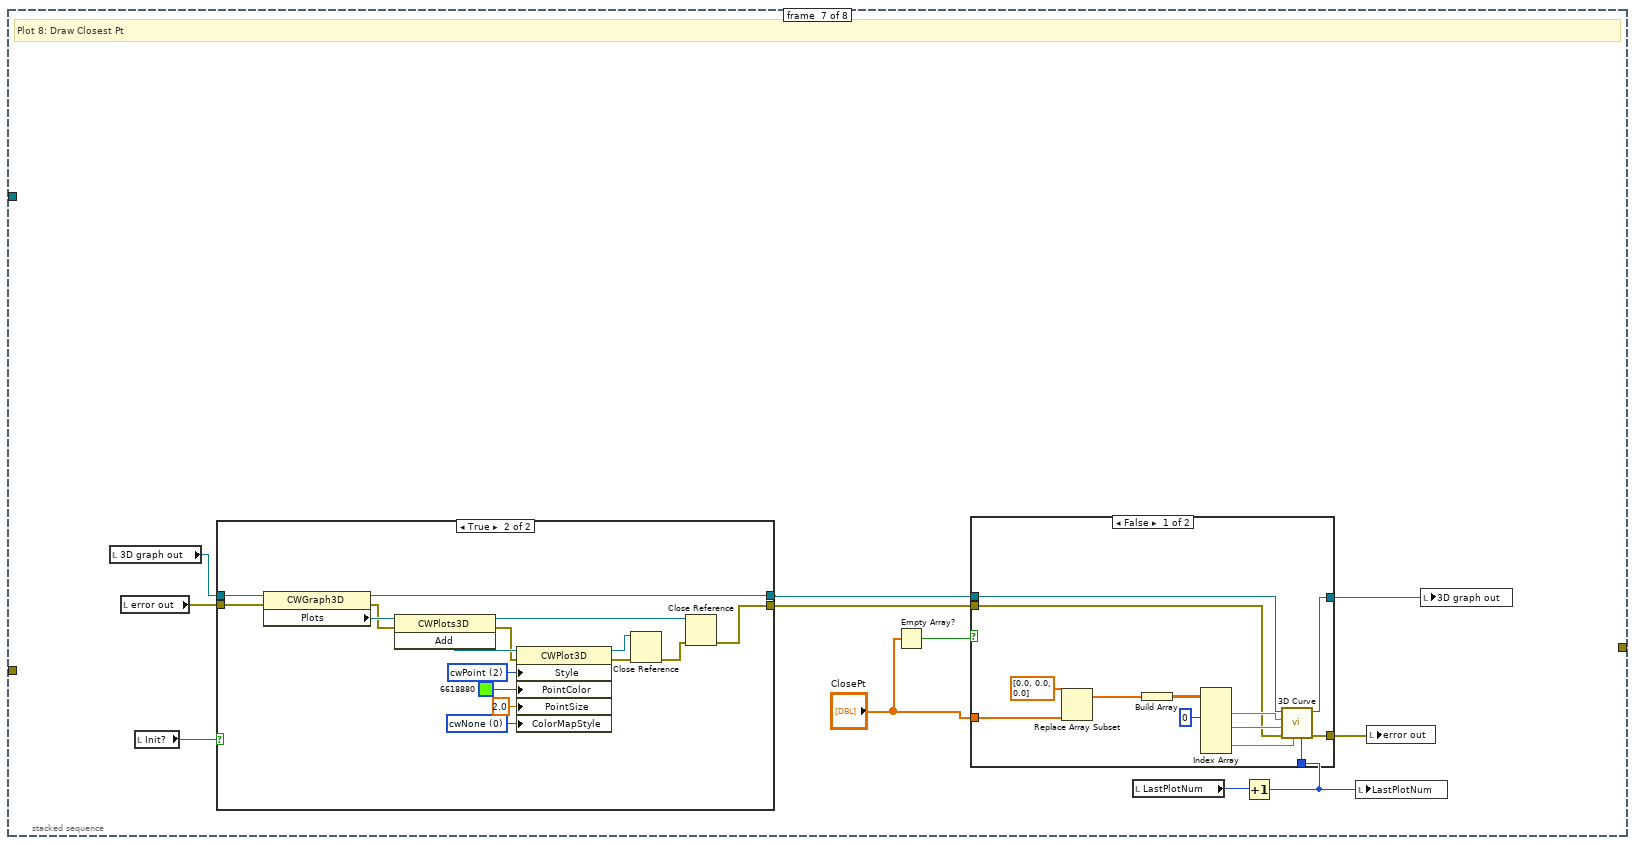
[diagram p17: hidden frame]
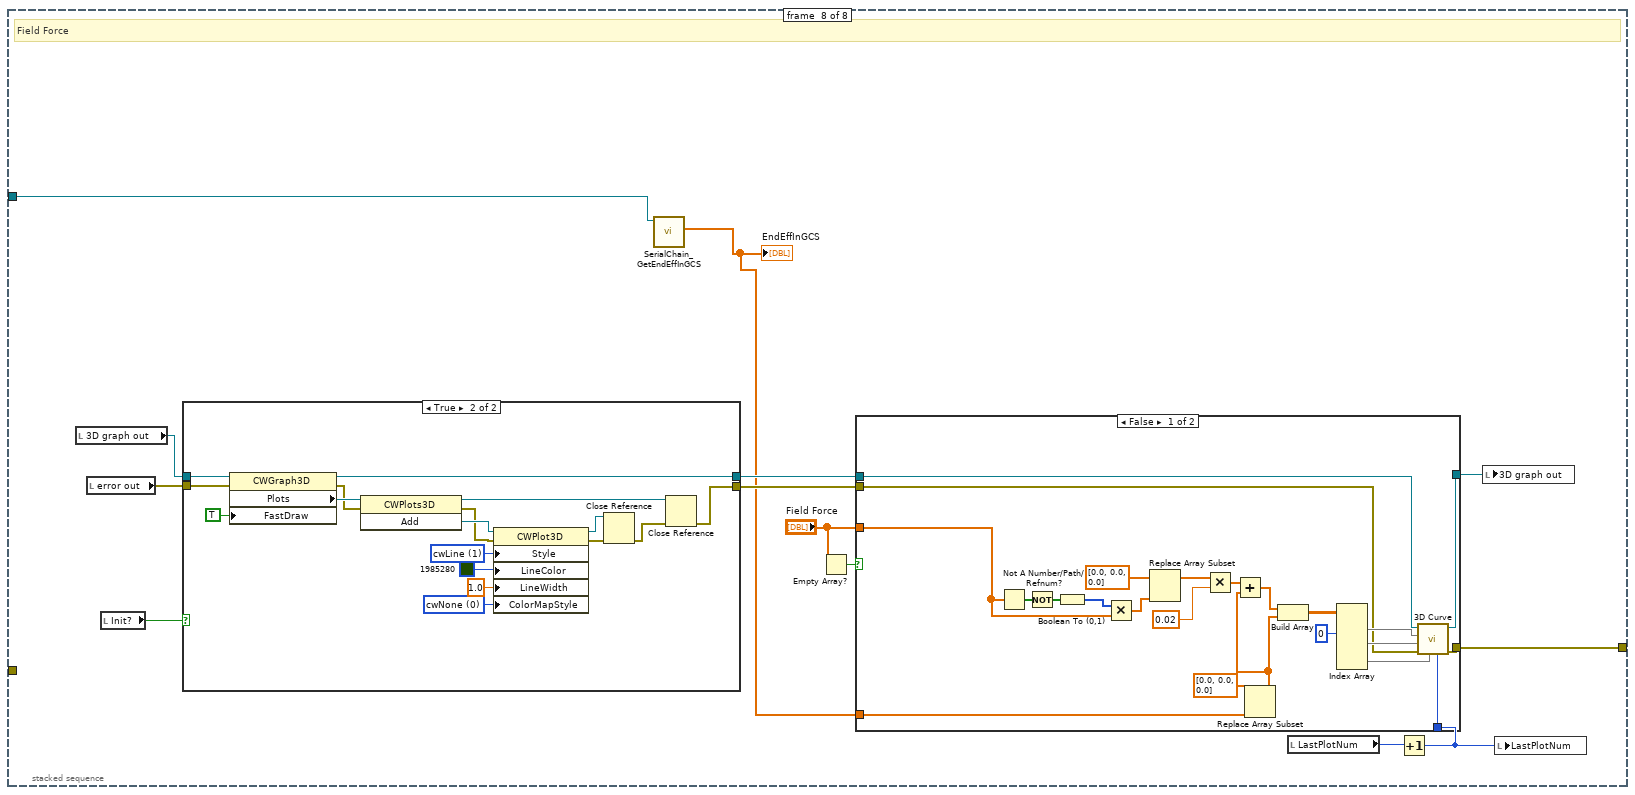
[diagram p20: hidden frame]
diagram:
  n1 = case shown="No Error" "error in (no error)" {
    selector: "error in (no error)" -> [w6 w379]
    tunnel: [w7 w379] -> w1
    tunnel: [w5 w378] -> w2
    tunnel: "CLX2 in" -> [w5 w378]
    frame No Error {
      n2 = stacked-sequence {
        tunnel: [_ _ _ _ _ _ _ w323] -> w7
        tunnel: w6 -> [_ w12 _ _ _ _ _ _]
        tunnel: w5 -> [_ _ w68 w104 _ w206 _ w322]
        frame #0 {
          n3 = First Call?() -> (First Call?: T/F=w10:bool)
          n4 = Or(x="Init?", y=w10) -> (x .or. y?=w8:bool)
          n5 = local write "Init?"(w8) -> ()
        }
        frame #1 {
          # "Initialized"
          n6 = local read "Init?"() -> (w11:bool)
          n7 = case shown="True" w11 {
            tunnel: "3D graph in" -> [w18 w32]
            tunnel: [w18 w28] -> w15
            tunnel: [w17 w23] -> w13
            tunnel: w12 -> [w17 w30]
            frame False {
            }
            frame True {
              n8 = invoke class="CWGraph3D" method="ClearData"(reference=w32, error in=w30) -> (reference out=w31:refnum<k7>, error out=w29:errorcluster)  [unwired: 1 in, 1 out]
              n9 = call <vilib>:"Set Plots.vi"("3D graph"=w31, "# of plots(1)"=0, "error in (no error)"=w29) -> ("3D graph out"=w33:refnum<k7>, "error out"=w24:errorcluster)  [unwired: 11 in]
              n10 = Unbundle By Name("AxisSetting") -> ("AxisLabel"=w21:string[], "AxisMax"=w20:dbl[], "AxisMin"=w19:dbl[])
              n11 = property class="CWGraph3D"(reference=w33, error in=w24) -> (reference out=w28:refnum<k7>, error out=w25:errorcluster, "Axes"=w34:refnum<k7>)
              n12 = for {
                shift-right: [w44] -> w26
                shift-left: w34 -> [w57]
                shift-right: [w45] -> w27
                shift-left: w25 -> [w42]
                tunnel: w21 -> [w38] mode=indexing
                tunnel: w20 -> [w37] mode=indexing
                tunnel: w19 -> [w36] mode=indexing
                i -> [w40]
                w41 = 0 items=["cwAxisTextFixed", "cwAxisTextFaceCamera"] ("CaptionOrientationStyle")
                # "Set Axis"
                n13 = Increment(x=w40) -> (x+1=w39:i32)
                n14 = invoke class="CWAxes3D" method="Item"(reference=w57, error in=w42, "Item"=w39) -> (reference out=w44:refnum<k7>, error out=w43:errorcluster, "Item"=w56:refnum<k7>)  [unwired: 1 in, 1 out]
                n15 = property class="CWAxis3D"(reference=w56, error in=w43, "Caption"=w38, "Maximum"=w37, "Minimum"=w36, "CaptionOrientationStyle"=w41) -> (reference out=w46:refnum<k7>, error out=w49:errorcluster, "Ticks"=w55:refnum<k7>)
                n16 = property class="CWTicks3D"(reference=w55, error in=w49, "MajorDivisions"=5, "MajorTicks"=TRUE, "MinorTicks"=FALSE, "AutoDivisions"=FALSE) -> (reference out=w48:refnum<k7>, error out=w50:errorcluster)
                n17 = Close Reference(reference=w48, error in (no error)=w50) -> (error out=w47:errorcluster)
                n18 = Close Reference(reference=w46, error in (no error)=w47) -> (error out=w45:errorcluster)
              }
              n19 = Close Reference(reference=w26, error in (no error)=w27) -> (error out=w23:errorcluster)
            }
          }
          "3D graph out" <- w15
          n20 = local write "error out"(w13) -> ()
          "LastPlotNum" <- 0 ("LastPlotNum 2")
        }
        frame #2 {
          # "Plot 1: Draw the leg"
          n21 = local read "error out"() -> (w60:errorcluster)
          n22 = local read "3D graph out"() -> (w66:refnum<k7>)
          n23 = call "SerialChain_GetJointCoordInGCS.vi"("error in (no error)"=w60, "SerialChain in"=w68) -> ("error out"=w59:errorcluster, "Joint Coord in GCS"=w58:dbl[][])  [unwired: 5 in, 3 out]
          n24 = local read "Init?"() -> (w62:bool)
          n25 = case shown="True" w62 {
            tunnel: w59 -> [w84 w97]
            tunnel: w66 -> [w85 w92]
            tunnel: [w85 w91] -> w65
            tunnel: [w84 w86] -> w64
            frame False {
            }
            frame True {
              w90 = 0 items=["cwNone", "cwShaded", "cwColorSpectrum", "cwGrayScale", "cwCustom"] ("ColorMapStyle")
              w103 = 3 items=["cwLine"=1, "cwPoint"=2, "cwLinePoint"=3, "cwHiddenLine"=4, "cwSurface"=5, "cwSurfaceLine"=6, "cwSurfaceNormal"=7, "cwContourLine"=8, "cwSurfaceContour"=9] ("Style")
              n26 = property class="CWGraph3D"(reference=w92, error in=w97) -> (reference out=w91:refnum<k7>, error out=w100:errorcluster, "Plots"=w101:refnum<k7>)
              n27 = invoke class="CWPlots3D" method="Add"(reference=w101, error in=w100) -> (reference out=w88:refnum<k7>, error out=w89:errorcluster, "Add"=w102:refnum<k7>)  [unwired: 1 in]
              n28 = property class="CWPlot3D"(reference=w102, error in=w89, "Style"=w103, "LineColor"=u32 16860, "LineWidth"=3.0, "PointColor"=u32 16744512, "PointSize"=3.0 ("LineWidth"), "ColorMapStyle"=w90) -> (reference out=w98:refnum<k7>, error out=w99:errorcluster)
              n29 = Close Reference(reference=w98, error in (no error)=w99) -> (error out=w87:errorcluster)
              n30 = Close Reference(reference=w88, error in (no error)=w87) -> (error out=w86:errorcluster)
            }
          }
          n31 = Empty Array?(array=w58) -> (empty?=w61:bool)
          n32 = local read "LastPlotNum"() -> (w70:i32)
          n33 = Increment(x=w70) -> (x+1=w69:i32)
          n34 = case shown="False" w61 {
            tunnel: [w76 w83] -> w67
            tunnel: w65 -> [w75 w83]
            tunnel: w64 -> [w74 w82]
            tunnel: [w73 w82] -> w63
            tunnel: w69 -> [w72 _]
            tunnel: w58 -> [w71 _]
            frame False {
              n35 = Transpose 2D Array(2D array=w71) -> (transposed array=w77:dbl[][])
              n36 = Index Array(array=w77, index (row) #1=0 ("index (row)")) -> (element #1=w79:dbl[], element #2=w80:dbl[], element #3=w81:dbl[])  [unwired: 5 in]
              n37 = call <vilib>:"3D Curve.vi"("plot number (1)"=w72, "z vector"=w81, "error in (no error)"=w74, "y vector"=w80, "x vector"=w79, "3D graph"=w75) -> ("error out"=w73:errorcluster, "3D graph out"=w76:refnum<k7>)  [unwired: 4 in]
            }
            frame True {
            }
          }
          n38 = local write "LastPlotNum"(w69) -> ()
          n39 = local write "3D graph out"(w67) -> ()
          n40 = local write "error out"(w63) -> ()
        }
        frame #3 {
          # "Plot 2: Draw the eff history"
          n41 = disable-structure shown="Disabled" {
            disable-tunnel: w104 -> [w117 _]
            frame Disabled {
              n42 = local read "3D graph out"() -> (w112:refnum<k7>)
              n43 = local read "error out"() -> (w113:errorcluster)
              n44 = local read "Init?"() -> (w109:bool)
              n45 = case shown="True" w109 {
                tunnel: w113 -> [w134 w147]
                tunnel: w112 -> [w135 w142]
                tunnel: [w135 w141] -> w111
                tunnel: [w134 w136] -> w106
                frame False {
                }
                frame True {
                  w140 = 0 items=["cwNone", "cwShaded", "cwColorSpectrum", "cwGrayScale", "cwCustom"] ("ColorMapStyle")
                  w154 = 1 items=["cwLine"=1, "cwPoint"=2, "cwLinePoint"=3, "cwHiddenLine"=4, "cwSurface"=5, "cwSurfaceLine"=6, "cwSurfaceNormal"=7, "cwContourLine"=8, "cwSurfaceContour"=9] ("Style")
                  n46 = property class="CWGraph3D"(reference=w142, error in=w147) -> (reference out=w141:refnum<k7>, error out=w151:errorcluster, "Plots"=w152:refnum<k7>)
                  n47 = invoke class="CWPlots3D" method="Add"(reference=w152, error in=w151) -> (reference out=w150:refnum<k7>, error out=w138:errorcluster, "Add"=w153:refnum<k7>)  [unwired: 1 in]
                  n48 = property class="CWPlot3D"(reference=w153, error in=w138, "Style"=w154, "LineColor"=u32 16744512, "LineWidth"=2.0, "PointColor"=u32 3381759, "PointSize"=2.0 ("LineWidth"), "ColorMapStyle"=w140, "Transparency"=50) -> (reference out=w148:refnum<k7>, error out=w149:errorcluster)
                  n49 = Close Reference(reference=w148, error in (no error)=w149) -> (error out=w137:errorcluster)
                  n50 = Close Reference(reference=w150, error in (no error)=w137) -> (error out=w136:errorcluster)
                }
              }
              n51 = local read "LastPlotNum"() -> (w115:i32)
              n52 = Increment(x=w115) -> (x+1=w116:i32)
              n53 = local write "LastPlotNum"(w116) -> ()
              n54 = Empty Array?(array=w107) -> (empty?=w108:bool)
              n55 = case shown="False" w108 {
                tunnel: [w131 w133] -> w114
                tunnel: w111 -> [w130 w133]
                tunnel: [w129 w132] -> w105
                tunnel: [w128 w132] -> w110
                tunnel: w116 -> [w127 _]
                tunnel: [w118 _] -> w107
                frame False {
                  n56 = Index Array(array=w118) -> (element #1=w124, element #2=w125, element #3=w126)  [unwired: 3 in]
                  n57 = local read "Init?"() -> (w119:bool)
                  n58 = call <vilib>:"Data Queue PtByPt.vi"("initialize"=w119, "sample length"="sample length", "input data point"=w125) -> ("Current Queue"=w121:dbl[])  [unwired: 4 in, 4 out]
                  n59 = call <vilib>:"Data Queue PtByPt.vi"("initialize"=w119, "sample length"="sample length", "input data point"=w126) -> ("Current Queue"=w120:dbl[])  [unwired: 4 in, 4 out]
                  n60 = call <vilib>:"Data Queue PtByPt.vi"("initialize"=w119, "sample length"="sample length", "input data point"=w124) -> ("Current Queue"=w122:dbl[])  [unwired: 4 in, 4 out]
                  n61 = call <vilib>:"3D Curve.vi"("plot number (1)"=w127, "z vector"=w120, "error in (no error)"=w129, "y vector"=w121, "x vector"=w122, "3D graph"=w130) -> ("error out"=w128:errorcluster, "3D graph out"=w131:refnum<k7>)  [unwired: 4 in]
                }
                frame True {
                }
              }
              n62 = local write "3D graph out"(w114) -> ()
              n63 = local write "error out"(w110) -> ()
            }
            frame Enabled {
            }
          }
        }
        frame #4 {
          # "Plot 3: Draw Desire Traj"
          n64 = local read "3D graph out"() -> (w161:refnum<k7>)
          n65 = local read "error out"() -> (w162:errorcluster)
          n66 = local read "Init?"() -> (w159:bool)
          n67 = case shown="True" w159 {
            tunnel: w162 -> [w179 w190]
            tunnel: w161 -> [w180 w187]
            tunnel: [w180 w186] -> w160
            tunnel: [w179 w181] -> w158
            frame False {
            }
            frame True {
              w184 = 0 items=["cwNone", "cwShaded", "cwColorSpectrum", "cwGrayScale", "cwCustom"] ("ColorMapStyle")
              w197 = 1 items=["cwLine"=1, "cwPoint"=2, "cwLinePoint"=3, "cwHiddenLine"=4, "cwSurface"=5, "cwSurfaceLine"=6, "cwSurfaceNormal"=7, "cwContourLine"=8, "cwSurfaceContour"=9] ("Style")
              n68 = property class="CWGraph3D"(reference=w187, error in=w190) -> (reference out=w186:refnum<k7>, error out=w194:errorcluster, "Plots"=w195:refnum<k7>)
              n69 = invoke class="CWPlots3D" method="Add"(reference=w195, error in=w194) -> (reference out=w193:refnum<k7>, error out=w183:errorcluster, "Add"=w196:refnum<k7>)  [unwired: 1 in]
              n70 = property class="CWPlot3D"(reference=w196, error in=w183, "Style"=w197, "LineColor"=u32 16744703, "LineWidth"=1.0, "Transparency"=0, "ColorMapStyle"=w184) -> (reference out=w191:refnum<k7>, error out=w192:errorcluster)
              n71 = Close Reference(reference=w191, error in (no error)=w192) -> (error out=w182:errorcluster)
              n72 = Close Reference(reference=w193, error in (no error)=w182) -> (error out=w181:errorcluster)
            }
          }
          n73 = Empty Array?(array="AnkleTraj_Target") -> (empty?=w156:bool)
          n74 = local read "LastPlotNum"() -> (w165:i32)
          n75 = Increment(x=w165) -> (x+1=w164:i32)
          n76 = case shown="False" w156 {
            tunnel: "AnkleTraj_Target" -> [w176 _]
            tunnel: [w170 w178] -> w163
            tunnel: w160 -> [w169 w178]
            tunnel: w164 -> [w168 _]
            tunnel: w158 -> [w167 w177]
            tunnel: [w166 w177] -> w157
            frame False {
              n77 = Transpose 2D Array(2D array=w176) -> (transposed array=w171:dbl[][])
              n78 = Index Array(array=w171, index (row) #1=0 ("index (row)")) -> (element #1=w173:dbl[], element #2=w174:dbl[], element #3=w175:dbl[])  [unwired: 5 in]
              n79 = call <vilib>:"3D Curve.vi"("plot number (1)"=w168, "z vector"=w175, "error in (no error)"=w167, "y vector"=w174, "x vector"=w173, "3D graph"=w169) -> ("error out"=w166:errorcluster, "3D graph out"=w170:refnum<k7>)  [unwired: 4 in]
            }
            frame True {
            }
          }
          n80 = local write "LastPlotNum"(w164) -> ()
          n81 = local write "3D graph out"(w163) -> ()
          n82 = local write "error out"(w157) -> ()
        }
        frame #5 {
          # "Plot 4~7: Draw Cables"
          n83 = local read "error out"() -> (w200:errorcluster)
          n84 = local read "LastPlotNum"() -> (w209:i32)
          n85 = local read "3D graph out"() -> (w204:refnum<k7>)
          n86 = local read "Init?"() -> (w199:bool)
          n87 = call "scc_GetCableInGCS.vi"("error in (no error)"=w200, "SerialChain_Cable in"=w206) -> ("error out"=w201:errorcluster, "Cable ID"=w198:i32[], "Cables Points"=w203:cluster{"PointInGCS":dbl[][]}[])  [unwired: 6 in, 1 out]
          n88 = Increment(x=w209) -> (x+1=w208:i32)
          n89 = for {
            tunnel: w203 -> [w227] mode=indexing
            shift-right: [w226] -> w205
            shift-left: w204 -> [w221]
            tunnel: w208 -> [w220]
            tunnel: [w219] -> w207
            shift-right: [w218] -> w202
            shift-left: w201 -> [w217]
            tunnel: w199 -> [w216]
            tunnel: w198 -> [w214] mode=indexing
            i -> [w222]
            w212 = 0 ("index (row)")
            n90 = Unbundle(w227) -> ("PointInGCS"=w213:dbl[][])
            n91 = Index Array(array=w213, index (row)=w212, index (col)=w212) -> (element=w211:dbl)
            n92 = case shown="True" w216 {
              tunnel: w217 -> [w230 w248]
              tunnel: w221 -> [w231 w242]
              tunnel: [w231 w237] -> w215
              tunnel: w214 -> [_ w239]
              tunnel: w211 -> [_ w238]
              tunnel: [w230 w232] -> w210
              frame False {
              }
              frame True {
                w243 = 0 items=["cwNone", "cwShaded", "cwColorSpectrum", "cwGrayScale", "cwCustom"] ("ColorMapStyle")
                w254 = 3 items=["cwLine"=1, "cwPoint"=2, "cwLinePoint"=3, "cwHiddenLine"=4, "cwSurface"=5, "cwSurfaceLine"=6, "cwSurfaceNormal"=7, "cwContourLine"=8, "cwSurfaceContour"=9] ("Style")
                n93 = property class="CWGraph3D"(reference=w242, error in=w248) -> (reference out=w237:refnum<k7>, error out=w235:errorcluster, "Plots"=w252:refnum<k7>, "Axes"=w236:refnum<k7>)
                n94 = disable-structure shown="Enabled" {
                  disable-tunnel: w239 -> [w268 _]
                  disable-tunnel: w238 -> [w266 _]
                  disable-tunnel: w236 -> [w265 _]
                  disable-tunnel: w235 -> [w264 w276]
                  disable-tunnel: [w255 w276] -> w234
                  frame Disabled {
                    n95 = Number To Decimal String(number=w268) -> (decimal integer string=w267:string)  [unwired: 1 in]
                    n96 = invoke class="CWAxes3D" method="Item"(reference=w265, error in=w264, "Item"=1) -> (reference out=w257:refnum<k7>, error out=w269:errorcluster, "Item"=w273:refnum<k7>)  [unwired: 1 in, 1 out]
                    n97 = property class="CWAxis3D"(reference=w273, error in=w269) -> (reference out=w259:refnum<k7>, error out=w270:errorcluster, "ValuePairs"=w275:refnum<k7>)
                    n98 = invoke class="CWValuePairs" method="Add"(reference=w275, error in=w270) -> (reference out=w261:refnum<k7>, error out=w271:errorcluster, "Add"=w272:refnum<k7>)  [unwired: 1 in]
                    n99 = property class="CWValuePair"(reference=w272, error in=w271, "Name"=w267, "Value"=w266) -> (reference out=w262:refnum<k7>, error out=w263:errorcluster)
                    n100 = Close Reference(reference=w262, error in (no error)=w263) -> (error out=w260:errorcluster)
                    n101 = Close Reference(reference=w261, error in (no error)=w260) -> (error out=w258:errorcluster)
                    n102 = Close Reference(reference=w259, error in (no error)=w258) -> (error out=w256:errorcluster)
                    n103 = Close Reference(reference=w257, error in (no error)=w256) -> (error out=w255:errorcluster)
                  }
                  frame Enabled {
                  }
                }
                n104 = invoke class="CWPlots3D" method="Add"(reference=w252, error in=w235) -> (reference out=w251:refnum<k7>, error out=w241:errorcluster, "Add"=w253:refnum<k7>)  [unwired: 1 in]
                n105 = property class="CWPlot3D"(reference=w253, error in=w241, "Style"=w254, "LineColor"=u32 13816530, "LineWidth"=0.0, "PointColor"=u32 6618880, "PointSize"=1.0 ("LineWidth"), "ColorMapStyle"=w243) -> (reference out=w249:refnum<k7>, error out=w250:errorcluster)
                n106 = Close Reference(reference=w249, error in (no error)=w250) -> (error out=w240:errorcluster)
                n107 = Close Reference(reference=w251, error in (no error)=w240) -> (error out=w233:errorcluster)
                n108 = Merge Errors(w233, w234) -> (w232:errorcluster)
              }
            }
            n109 = Add(x=w222, y=w220) -> (x+y=w219:i32)
            n110 = Transpose 2D Array(2D array=w213) -> (transposed array=w228:dbl[][])
            n111 = Index Array(array=w228, index (row) #1=0 ("index (row)")) -> (element #1=w225:dbl[], element #2=w224:dbl[], element #3=w223:dbl[])  [unwired: 5 in]
            n112 = call <vilib>:"3D Curve.vi"("plot number (1)"=w219, "z vector"=w223, "error in (no error)"=w210, "y vector"=w224, "x vector"=w225, "3D graph"=w215) -> ("error out"=w218:errorcluster, "3D graph out"=w226:refnum<k7>)  [unwired: 4 in]
          }
          n113 = local write "error out"(w202) -> ()
          n114 = local write "3D graph out"(w205) -> ()
          n115 = local write "LastPlotNum"(w207) -> ()
        }
        frame #6 {
          # "Plot 8: Draw Closest Pt"
          n116 = local read "3D graph out"() -> (w285:refnum<k7>)
          n117 = local read "error out"() -> (w286:errorcluster)
          n118 = local read "Init?"() -> (w284:bool)
          n119 = case shown="True" w284 {
            tunnel: w286 -> [w303 w313]
            tunnel: w285 -> [w304 w310]
            tunnel: [w304 w309] -> w283
            tunnel: [w303 w305] -> w280
            frame False {
            }
            frame True {
              w308 = 0 items=["cwNone", "cwShaded", "cwColorSpectrum", "cwGrayScale", "cwCustom"] ("ColorMapStyle")
              w320 = 2 items=["cwLine"=1, "cwPoint"=2, "cwLinePoint"=3, "cwHiddenLine"=4, "cwSurface"=5, "cwSurfaceLine"=6, "cwSurfaceNormal"=7, "cwContourLine"=8, "cwSurfaceContour"=9] ("Style")
              n120 = property class="CWGraph3D"(reference=w310, error in=w313) -> (reference out=w309:refnum<k7>, error out=w317:errorcluster, "Plots"=w318:refnum<k7>)
              n121 = invoke class="CWPlots3D" method="Add"(reference=w318, error in=w317) -> (reference out=w316:refnum<k7>, error out=w307:errorcluster, "Add"=w319:refnum<k7>)  [unwired: 1 in]
              n122 = property class="CWPlot3D"(reference=w319, error in=w307, "Style"=w320, "PointColor"=u32 6618880, "PointSize"=2.0 ("LineWidth"), "ColorMapStyle"=w308) -> (reference out=w314:refnum<k7>, error out=w315:errorcluster)
              n123 = Close Reference(reference=w314, error in (no error)=w315) -> (error out=w306:errorcluster)
              n124 = Close Reference(reference=w316, error in (no error)=w306) -> (error out=w305:errorcluster)
            }
          }
          n125 = Empty Array?(array="ClosePt") -> (empty?=w277:bool)
          n126 = local read "LastPlotNum"() -> (w282:i32)
          n127 = Increment(x=w282) -> (x+1=w281:i32)
          n128 = case shown="False" w277 {
            tunnel: "ClosePt" -> [w299 _]
            tunnel: [w292 w302] -> w287
            tunnel: w283 -> [w291 w302]
            tunnel: w281 -> [w290 _]
            tunnel: w280 -> [w289 w301]
            tunnel: [w288 w301] -> w279
            frame False {
              n129 = Replace Array Subset(array=dbl[] [0.0, 0.0, 0.0], new element=w299) -> (w298:dbl[])  [unwired: 1 in]
              n130 = Build Array(w298) -> (w297:dbl[][])
              n131 = Index Array(array=w297, index (col) #1=0 ("disabled index (col)")) -> (element #1=w295:dbl[], element #2=w294:dbl[], element #3=w293:dbl[])  [unwired: 5 in]
              n132 = call <vilib>:"3D Curve.vi"("plot number (1)"=w290, "z vector"=w293, "error in (no error)"=w289, "y vector"=w294, "x vector"=w295, "3D graph"=w291) -> ("error out"=w288:errorcluster, "3D graph out"=w292:refnum<k7>)  [unwired: 4 in]
            }
            frame True {
            }
          }
          n133 = local write "LastPlotNum"(w281) -> ()
          n134 = local write "error out"(w279) -> ()
          n135 = local write "3D graph out"(w287) -> ()
        }
        frame #7 {
          # "Field Force"
          n136 = local read "3D graph out"() -> (w331:refnum<k7>)
          n137 = local read "error out"() -> (w332:errorcluster)
          n138 = local read "Init?"() -> (w330:bool)
          n139 = case shown="True" w330 {
            tunnel: w332 -> [w359 w370]
            tunnel: w331 -> [w360 w367]
            tunnel: [w360 w366] -> w329
            tunnel: [w359 w361] -> w326
            frame False {
            }
            frame True {
              w365 = 0 items=["cwNone", "cwShaded", "cwColorSpectrum", "cwGrayScale", "cwCustom"] ("ColorMapStyle")
              w377 = 1 items=["cwLine"=1, "cwPoint"=2, "cwLinePoint"=3, "cwHiddenLine"=4, "cwSurface"=5, "cwSurfaceLine"=6, "cwSurfaceNormal"=7, "cwContourLine"=8, "cwSurfaceContour"=9] ("Style")
              n140 = property class="CWGraph3D"(reference=w367, error in=w370, "FastDraw"=TRUE) -> (reference out=w366:refnum<k7>, error out=w374:errorcluster, "Plots"=w375:refnum<k7>)
              n141 = invoke class="CWPlots3D" method="Add"(reference=w375, error in=w374) -> (reference out=w373:refnum<k7>, error out=w363:errorcluster, "Add"=w376:refnum<k7>)  [unwired: 1 in]
              n142 = property class="CWPlot3D"(reference=w376, error in=w363, "Style"=w377, "LineColor"=u32 1985280, "LineWidth"=1.0, "ColorMapStyle"=w365) -> (reference out=w371:refnum<k7>, error out=w372:errorcluster)
              n143 = Close Reference(reference=w371, error in (no error)=w372) -> (error out=w362:errorcluster)
              n144 = Close Reference(reference=w373, error in (no error)=w362) -> (error out=w361:errorcluster)
            }
          }
          n145 = call "SerialChain_GetEndEffInGCS.vi"("SerialChain in"=w322) -> ("Pendeff(GCS)"=w321:dbl[])  [unwired: 6 in, 4 out]
          "EndEffInGCS" <- w321
          n146 = Empty Array?(array="Field Force") -> (empty?=w324:bool)
          n147 = local read "LastPlotNum"() -> (w328:i32)
          n148 = Increment(x=w328) -> (x+1=w327:i32)
          n149 = case shown="False" w324 {
            tunnel: [w340 w358] -> w333
            tunnel: w329 -> [w339 w358]
            tunnel: w327 -> [w338 _]
            tunnel: w326 -> [w337 w357]
            tunnel: [w336 w357] -> w323
            tunnel: "Field Force" -> [w335 _]
            tunnel: w321 -> [w334 _]
            frame False {
              n150 = Not A Number/Path/Refnum?(number/path/refnum=w335) -> (NaN/Path/Refnum?=w344:bool[])
              n151 = Not(x=w344) -> (.not. x?=w343:bool[])
              n152 = Boolean To (0,1)(Boolean=w343) -> (0, 1=w342:i16[])
              n153 = Multiply(x=w342, y=w335) -> (x*y=w341:dbl[])
              n154 = Replace Array Subset(array=dbl[] [0.0, 0.0, 0.0], new element=w341) -> (w354:dbl[])  [unwired: 1 in]
              n155 = Multiply(x=w354, y=0.02) -> (x*y=w349:dbl[])
              n156 = Replace Array Subset(array=dbl[] [0.0, 0.0, 0.0], new element=w334) -> (w356:dbl[])  [unwired: 1 in]
              n157 = Add(x=w349, y=w356) -> (x+y=w346:dbl[])
              n158 = Build Array(w346, w356) -> (w347:dbl[][])
              n159 = Index Array(array=w347, index (col) #1=0 ("disabled index (col)")) -> (element #1=w350:dbl[], element #2=w351:dbl[], element #3=w352:dbl[])  [unwired: 5 in]
              n160 = call <vilib>:"3D Curve.vi"("plot number (1)"=w338, "z vector"=w352, "error in (no error)"=w337, "y vector"=w351, "x vector"=w350, "3D graph"=w339) -> ("error out"=w336:errorcluster, "3D graph out"=w340:refnum<k7>)  [unwired: 4 in]
            }
            frame True {
            }
          }
          n161 = local write "3D graph out"(w333) -> ()
          n162 = local write "LastPlotNum"(w327) -> ()
        }
      }
    }
    frame Error {
    }
  }
  "CLX2 out" <- w2
  "error out" <- w1
